vi "Configure Parameter to Measure.vi"(8 "error in (no error)":errorcluster, 10 "Sparameters (string)":string[](array[string]), 11 "VNA-ZNB in":refnum<class "VNA-ZNB.lvclass">) -> (0 "error out":errorcluster, 3 "VNA-ZNB out":refnum<class "VNA-ZNB.lvclass">)   [LabVIEW 2020, in "VNA-ZNB.lvclass"]
uses:
  VNA-ZNB.lvclass
  Vector Network Analyzer.lvclass
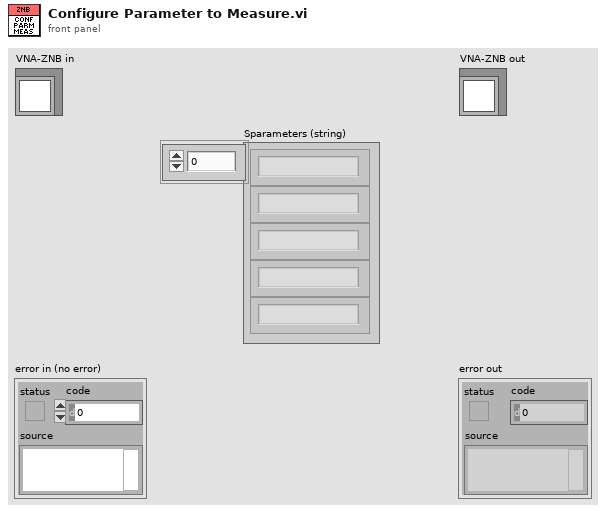
[diagram p1: front panel]
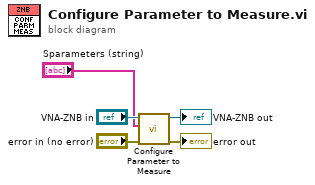
[diagram p0: block diagram]
diagram:
  n1 = call-parent "Configure Parameter to Measure.vi"("error in (no error)"="error in (no error)", "Sparameters (string)"="Sparameters (string)", "Vector Network Analyzer in"="VNA-ZNB in") -> ("error out"=→"error out":errorcluster, "Vector Network Analyzer out"=→"VNA-ZNB out":refnum<class "VNA-ZNB.lvclass">)  [unwired: 7 in]
